vi "Is Overhaul.vi"(8 "overhaul in":bool, 9 "goal node in":refnum<data-value>, 10 "current node in":refnum<data-value>, 11 "RVCLibrary_Bug2 in":refnum<class "RVCLibrary_Bug2.lvclass">) -> (0 "overhaul out":bool, 1 "goal node out":refnum<data-value>, 2 "current node out":refnum<data-value>, 3 "RVCLibrary_Bug2 out":refnum<class "RVCLibrary_Bug2.lvclass">)   [LabVIEW 2013, in "RVCLibrary_Bug2.lvclass"]
uses:
  RVCLibrary_Bug2.lvclass
  <vilib>/robotics/Navigation/shared/MapNode/AbstractDstarNode/NI_Robotics_AbstractDstarNode.lvclass
  RVCLibrary_Bug2.lvclass/RVCLibrary_Bug2.ctl
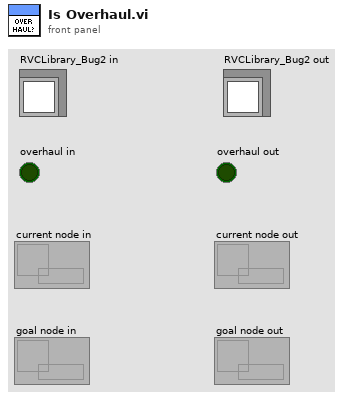
[diagram p1: front panel]
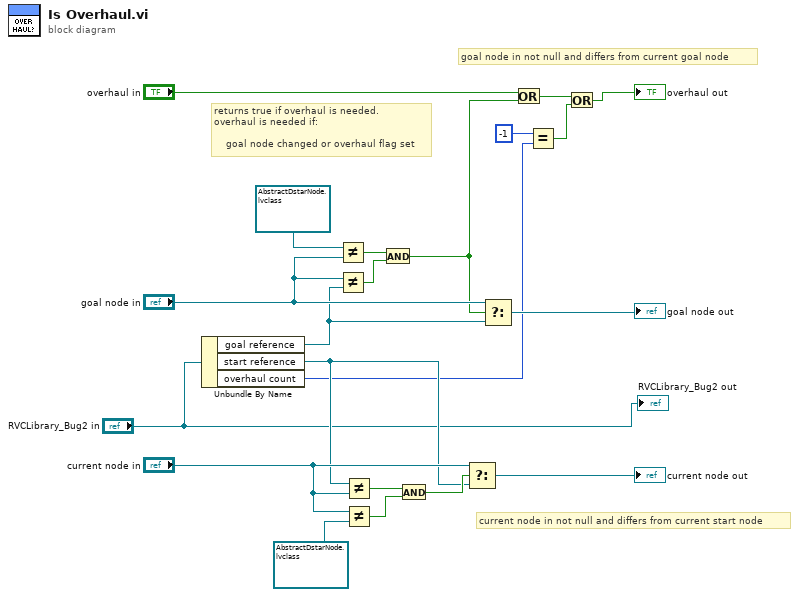
[diagram p0: block diagram]
diagram:
  # "returns true if overhaul is needed.\noverhaul is needed if:\n\n    goal node changed or overhaul flag set"
  # "current node in not null and differs from current start node"
  # "goal node in not null and differs from current goal node"
  n1 = Unbundle By Name("RVCLibrary_Bug2 in") -> ("goal reference"=w8:refnum<data-value>, "start reference"=w15:refnum<data-value>, "overhaul count"=w6:i32)
  n2 = Not Equal?(x=refnum<data-value> refnum ("node in"), y="goal node in") -> (x != y?=w12:bool)
  n3 = Not Equal?(x="goal node in", y=w8) -> (x != y?=w11:bool)
  n4 = Not Equal?(x=w15, y="current node in") -> (x != y?=w18:bool)
  n5 = Not Equal?(x="current node in", y=refnum<data-value> refnum ("node in")) -> (x != y?=w19:bool)
  n6 = And(x=w12, y=w11) -> (x .and. y?=w7:bool)
  n7 = And(x=w18, y=w19) -> (x .and. y?=w17:bool)
  n8 = Select(t="current node in", s=w17, f=w15) -> (s? t:f=→"current node out":refnum<data-value>)
  n9 = Select(t="goal node in", s=w7, f=w8) -> (s? t:f=→"goal node out":refnum<data-value>)
  n10 = Or(x="overhaul in", y=w7) -> (x .or. y?=w4:bool)
  n11 = Equal?(x=-1, y=w6) -> (x = y?=w3:bool)
  n12 = Or(x=w4, y=w3) -> (x .or. y?=→"overhaul out":bool)
  "RVCLibrary_Bug2 out" <- "RVCLibrary_Bug2 in"
